vi "Save-Load Last used profile name.vi"(8 "error in":errorcluster, 11 "Function":T1=enum."Load from file") -> (0 "error out":errorcluster, 2 "Name of last profile saved":string, 3 "Last used profile for selected user":string)   [LabVIEW 2013]
uses:
  Typedefs/Save-Load enum.ctl
  Typedefs/Which path.ctl
  <vilib>/Utility/config.llb/NI_LVConfig.lvlib
panel:
  out "User Name":string
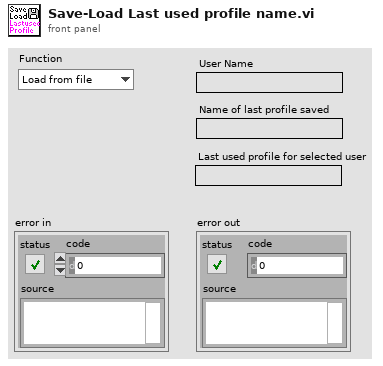
[diagram p1: front panel]
types:
  T1 = typedef "Save-Load enum.ctl" = enum16{"Save to file", "Load from file", "Compare from file"}
  T2 = typedef "Which path.ctl" = enum16{"Configuration Files", "Calibration Files", "Images", "Setup.ini", "Loaded User profile.ini", "User's-Previous session.ini", "New user profile.ini", "Selected User profile.ini", "User profiles folder", "Power meter scaling.txt", "FOV Cal.ini"}
  T3 = cluster{"key":string, "Save?":bool, "Default":string}
  T4 = cluster{"key":string, "Save?":bool, "Default":string}[]
  T5 = typedef "NI_LVConfig.lvlib/Config Data RefNum.ctl" = refnum<k1>
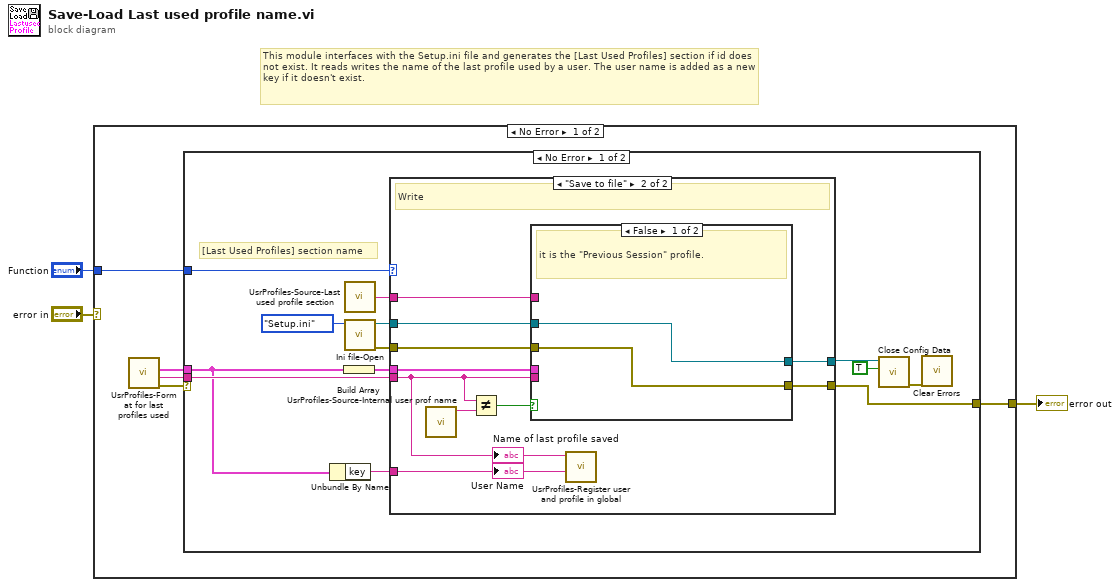
[diagram p0: block diagram]
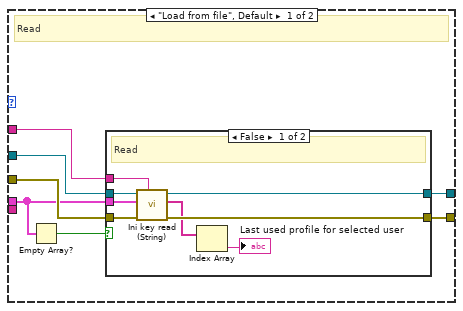
[diagram p2: hidden frame]
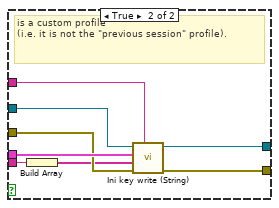
[diagram p4: hidden frame]
diagram:
  # "This module interfaces with the Setup.ini file and generates the [Last Used Profiles] section if id does not exist. It reads writes the name of the last profile used by a user. The user name is added as a new key if it doesn't exist."
  n1 = case shown="No Error" "error in" {
    selector: "error in" -> [_ w59]
    tunnel: [w8 w59] -> w3
    tunnel: "Function" -> [w5 _]
    frame No Error {
      n2 = call "UsrProfiles-Format for last profiles used.vi"() -> ("error out"=w4:errorcluster, "Selected profile name"=w6:string, "Key setup"=w7:T3)  [unwired: 9 in]
      n3 = case shown="No Error" w4 {
        tunnel: [w15 _] -> w8
        tunnel: w7 -> [w10 _]
        tunnel: w6 -> [w14 _]
        tunnel: w5 -> [w13 _]
        frame No Error {
          # "[Last Used Profiles] section name"
          n4 = Unbundle By Name(w10) -> ("key"=w9:string)
          n5 = Build Array(w10) -> (w12:T4)
          n6 = call "UsrProfiles-Source-Last used profile section.vi"() -> ("Last Used Profile section name"=w11:string)  [unwired: 1 in]
          n7 = call "Ini file-Open.vi"("Which file?"=Which_path."Setup.ini") -> ("error out"=w19:errorcluster, "User profile ini file ref"=w20:T5)  [unwired: 7 in, 2 out]
          n8 = case shown="\"Save to file\"" w13 {
            tunnel: [w24 w46] -> w15
            tunnel: [w23 w44] -> w18
            tunnel: w19 -> [w25 w43]
            tunnel: w20 -> [w26 w45]
            tunnel: w11 -> [w27 w48]
            tunnel: w14 -> [_ w41]
            tunnel: w12 -> [w22 w47]
            tunnel: w9 -> [_ w39]
            frame "Load from file", Default {
              # "Read"
              n9 = Empty Array?(array=w22) -> (empty?=w28:bool)
              n10 = case shown="False" w28 {
                tunnel: [w33 w38] -> w23
                tunnel: [w32 w37] -> w24
                tunnel: w22 -> [w35 _]
                tunnel: w26 -> [w36 w38]
                tunnel: w25 -> [w31 w37]
                tunnel: w27 -> [w34 _]
                frame False {
                  # "Read"
                  n11 = call "Ini key read (String).vi"("Section name"=w34, "error in (no error)"=w31, "Keys setup"=w35, "Ini file ref in"=w36) -> ("error out"=w32:errorcluster, "Value read/used"=w30:string[], "Ini file ref"=w33:T5)  [unwired: 5 in]
                  n12 = Index Array(array=w30) -> (element=→"Last used profile for selected user":string)  [unwired: 1 in]
                }
                frame True {
                  # "No parametersof such type"
                }
              }
            }
            frame "Save to file" {
              # "Write"
              n13 = call "UsrProfiles-Source-Internal user prof name.vi"() -> ("Previous session profile name"=w42:string)  [unwired: 11 in]
              n14 = Not Equal?(x=w41, y=w42) -> (x != y?=w40:bool)
              n15 = case shown="False" w40 {
                tunnel: w48 -> [_ w58]
                tunnel: w47 -> [_ w57]
                tunnel: [w49 w56] -> w46
                tunnel: w45 -> [w50 w55]
                tunnel: [w50 w54] -> w44
                tunnel: w43 -> [w49 w53]
                tunnel: w41 -> [_ w51]
                frame False {
                  # "it is the \"Previous Session\" profile."
                }
                frame True {
                  # "is a custom profile\n(i.e. it is not the \"previous session\" profile)."
                  n16 = Build Array(w51) -> (w52:string[])
                  n17 = call "Ini key write (String).vi"("Section"=w58, "error in (no error)"=w53, "Values (String)"=w52, "Ini file interface"=w57, "Ini file refnum in"=w55) -> ("error out"=w56:errorcluster, "Ini file refnum out"=w54:T5)  [unwired: 5 in]
                }
              }
              n18 = call "UsrProfiles-Register user and profile in global.vi"("User Name"=w39, "Profile name (no user prefix or file extension)"=w41) -> ()  [unwired: 9 in, 1 out]
              "Name of last profile saved" <- w41
              "User Name" <- w39
            }
          }
          n19 = call <vilib>:"Close Config Data.vi"("write file if changed (T)"=TRUE ("write configuration file? (F)"), "refnum"=w18) -> ("error out"=w17:errorcluster)  [unwired: 8 in, 1 out]
          n20 = call <vilib>:"Clear Errors.vi"("error in (no error)"=w17) -> ()  [unwired: 6 in, 1 out]
        }
        frame Error {
          # "This executes during software shutdown, if the Live imaging window was not opened during this session."
        }
      }
    }
    frame Error {
    }
  }
  "error out" <- w3
